vi "VI Name.vi"(8 "error in (no error)":errorcluster, 11 "Level (1)":i32=1) -> (0 "error out":errorcluster, 3 "VI Name":string)   [LabVIEW 2019, in "Unit Test Engine Tools.lvlib"]
uses:
  Unit Test Engine Tools.lvlib
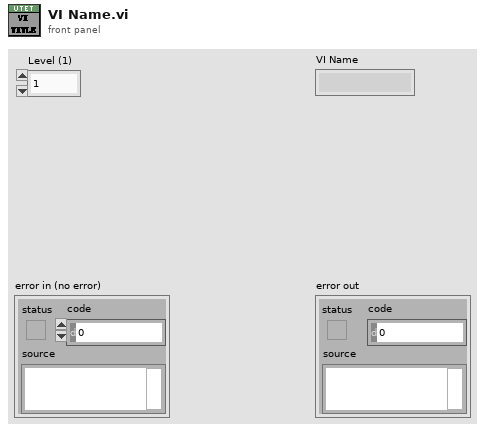
[diagram p1: front panel]
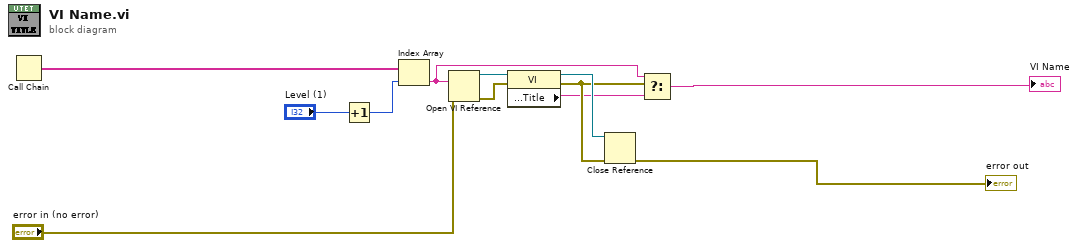
[diagram p0: block diagram]
diagram:
  n1 = Call Chain() -> (call chain=w9:string[])
  n2 = Increment(x="Level (1)") -> (x+1=w2:i32)
  n3 = Index Array(array=w9, index=w2) -> (element=w7:string)
  n4 = Open VI Reference(vi path=w7, error in (no error)="error in (no error)") -> (vi reference=w12:refnum<vi>, error out=w11:errorcluster)  [unwired: 4 in]
  n5 = property class="VI"(reference=w12, error in=w11) -> (reference out=w10:refnum<vi>, error out=w8:errorcluster, "Front Panel Window:Title"=w6:string)
  n6 = Close Reference(reference=w10, error in (no error)=w8) -> (error out=→"error out":errorcluster)
  n7 = Select(t=w7, s=w8, f=w6) -> (s? t:f=→"VI Name":string)
